vi "Top Level FPGA_w8randLED.vi"() -> ()   [LabVIEW 2012]
uses:
  <vilib>/Platform/TimedLoop/XDataNode/timing_clust.ctl
  <vilib>/Platform/TimedLoop/XDataNode/nitl_modes.ctl
  <vilib>/Platform/TimedLoop/XDataNode/wakeup.ctl
  <vilib>/rvi/DataTransferAndStorage/Container/Common/niFpgaContainerMetaDataKey.ctl
  <vilib>/rvi/DataTransferAndStorage/Container/Common/niFpgaContainerState.ctl
  <vilib>/rvi/DataTransferAndStorage/Container/Common/niFpgaDataTypeControl.ctl
  <vilib>/rvi/DataTransferAndStorage/Container/Common/niFpgaContainerImplementationControl.ctl
  <vilib>/rvi/DataTransferAndStorage/Container/Common/niFpgaContainerArbitrationOptionsControl.ctl
  <vilib>/rvi/DataTransferAndStorage/Container/Common/niFpgaTransferTypeControl.ctl
  <vilib>/rvi/DataTransferAndStorage/Container/Common/niFpgaContainerInitializationParameters.ctl
  <vilib>/rvi/Memory/Memory_Types/niFpgaMemoryInterfaceConfiguration.ctl
  <vilib>/rvi/FIFO/Fifo_Types/niFpgaFifoControlLogicControl.ctl
  <vilib>/rvi/eio/common/nirviEmuTemplateMethod_errors.vi
  <vilib>/rvi/FIFO/Fifo_Resource/nirvififoEmulationSetSize.vi
  <vilib>/rvi/DataTransferAndStorage/Container/Common/niFpgaContainerGetUniqueNameForEmu.vi
  <vilib>/rvi/Emulation/niFpgaSctlEmulationRegisterWithScheduler.vi
  <vilib>/rvi/DataTransferAndStorage/Container/Common/niFpgaContainerSetEmuInfo.vi
  <vilib>/rvi/eio/common/nirviEmuReportErrorAndStop.vi
  <vilib>/rvi/Emulation/niFpgaSctlEmulationScheduler.vi
  <vilib>/rvi/Emulation/niFpgaSctlEmulationFifoFullMgr.vi
  <vilib>/rvi/errors/niFpgaSetErrorForExecOnDevCompSimple.vi
  <vilib>/rvi/Memory/Memory_Emulation/nirvimemoryEmulationManagerCache_GetValue.vi
  <vilib>/rvi/Memory/Memory_Emulation/niFpgaMemoryEmulationValidateCache.vi
  <vilib>/rvi/Memory/Memory_Emulation/nirvimemoryEmulationManagerCache_InsertValue.vi
  <vilib>/rvi/Memory/Memory_Emulation/nirvimemoryEmulationManagerCache_SetValue.vi
  <vilib>/rvi/Emulation/niFpgaSctlEmulationResourceMgr.vi
  <vilib>/rvi/Memory/Memory_Emulation/niFpgaMemoryEmulationCacheClearOnFirstRun.vi
  <vilib>/rvi/Memory/Memory_Emulation/nirvimemoryEmulationManagerCache_MakeExclusive.vi
  <vilib>/rvi/Memory/Memory_Emulation/nirvimemoryEmulationManagerCache_ReleaseExclusive.vi
  <vilib>/Utility/error.llb/Clear Errors.vi
  <vilib>/eio/EIONode/EIONode.xnode
  <vilib>/rvi/DataTransferAndStorage/Container/XNode/niFpgaContainer.xnode
  <vilib>/rvi/FIFO/Fifo_Resource/nirvififoEmulationClear.vi
  <vilib>/Platform/TimedLoop/XDataNode/XDataNode.xnode
  <vilib>/rvi/LocalResourceManager/LocalResourceManager.xnode
  <vilib>/rvi/FIFO/Fifo_Resource/nirvififoEmulationRead.vi
  <vilib>/rvi/DataTransferAndStorage/Register/Emulation/niFpgaRegisterEmulation.vi
  <vilib>/rvi/Memory/Memory_Emulation/nirvimemoryEmulation.vi
  <vilib>/rvi/FIFO/Fifo_Resource/nirvififoEmulationWrite.vi
  <vilib>/Platform/TimedLoop/XDataNode/XDNodeRunTimeDep.lvlib
panel:
  in  "location":i16(ring) items=["Purdue", "NIKHEF", "Zurich", "???"]
  in  "Testpulse duration (20 ns ticks)":u32
  in  "initial value":u64
  in  "channel 7 on/off":bool
  in  "channel 6 on/off":bool
  in  "channel 5 on/off":bool
  in  "channel 4 on/off":bool
  in  "channel 3 on/off":bool
  in  "channel 1 on/off":bool
  in  "channel 2 on/off":bool
  in  "channel 0 on/off":bool
  out "Timestamp":u64
  in  "Stop FPGA and exit":bool
  out "DMA FIFO Timed Out?":bool
  in  "Testpulser On/Off":bool
  in  "Testpulse Time Delay (20 ns ticks)":u32=15
  in  "circular buffer length":u32=1000
  in  "# of pretrigger":u32=20
  out "IO Module\\Pll Unlocked":bool
  out "IO Module\\ADC Error B":bool
  out "IO Module\\ADC Error A":bool
  out "Init Done":bool
  in  "Trigger 4":i16=4000
  in  "Trigger 5":i16=4000
  in  "Trigger 6":i16=4000
  in  "Trigger 7":i16=4000
  in  "Trigger 2":i16=4000
  in  "Trigger 3":i16=4000
  in  "Trigger 1":i16=4000
  in  "Record Size only data":u32=95
  in  "Trigger 0":i16=4000
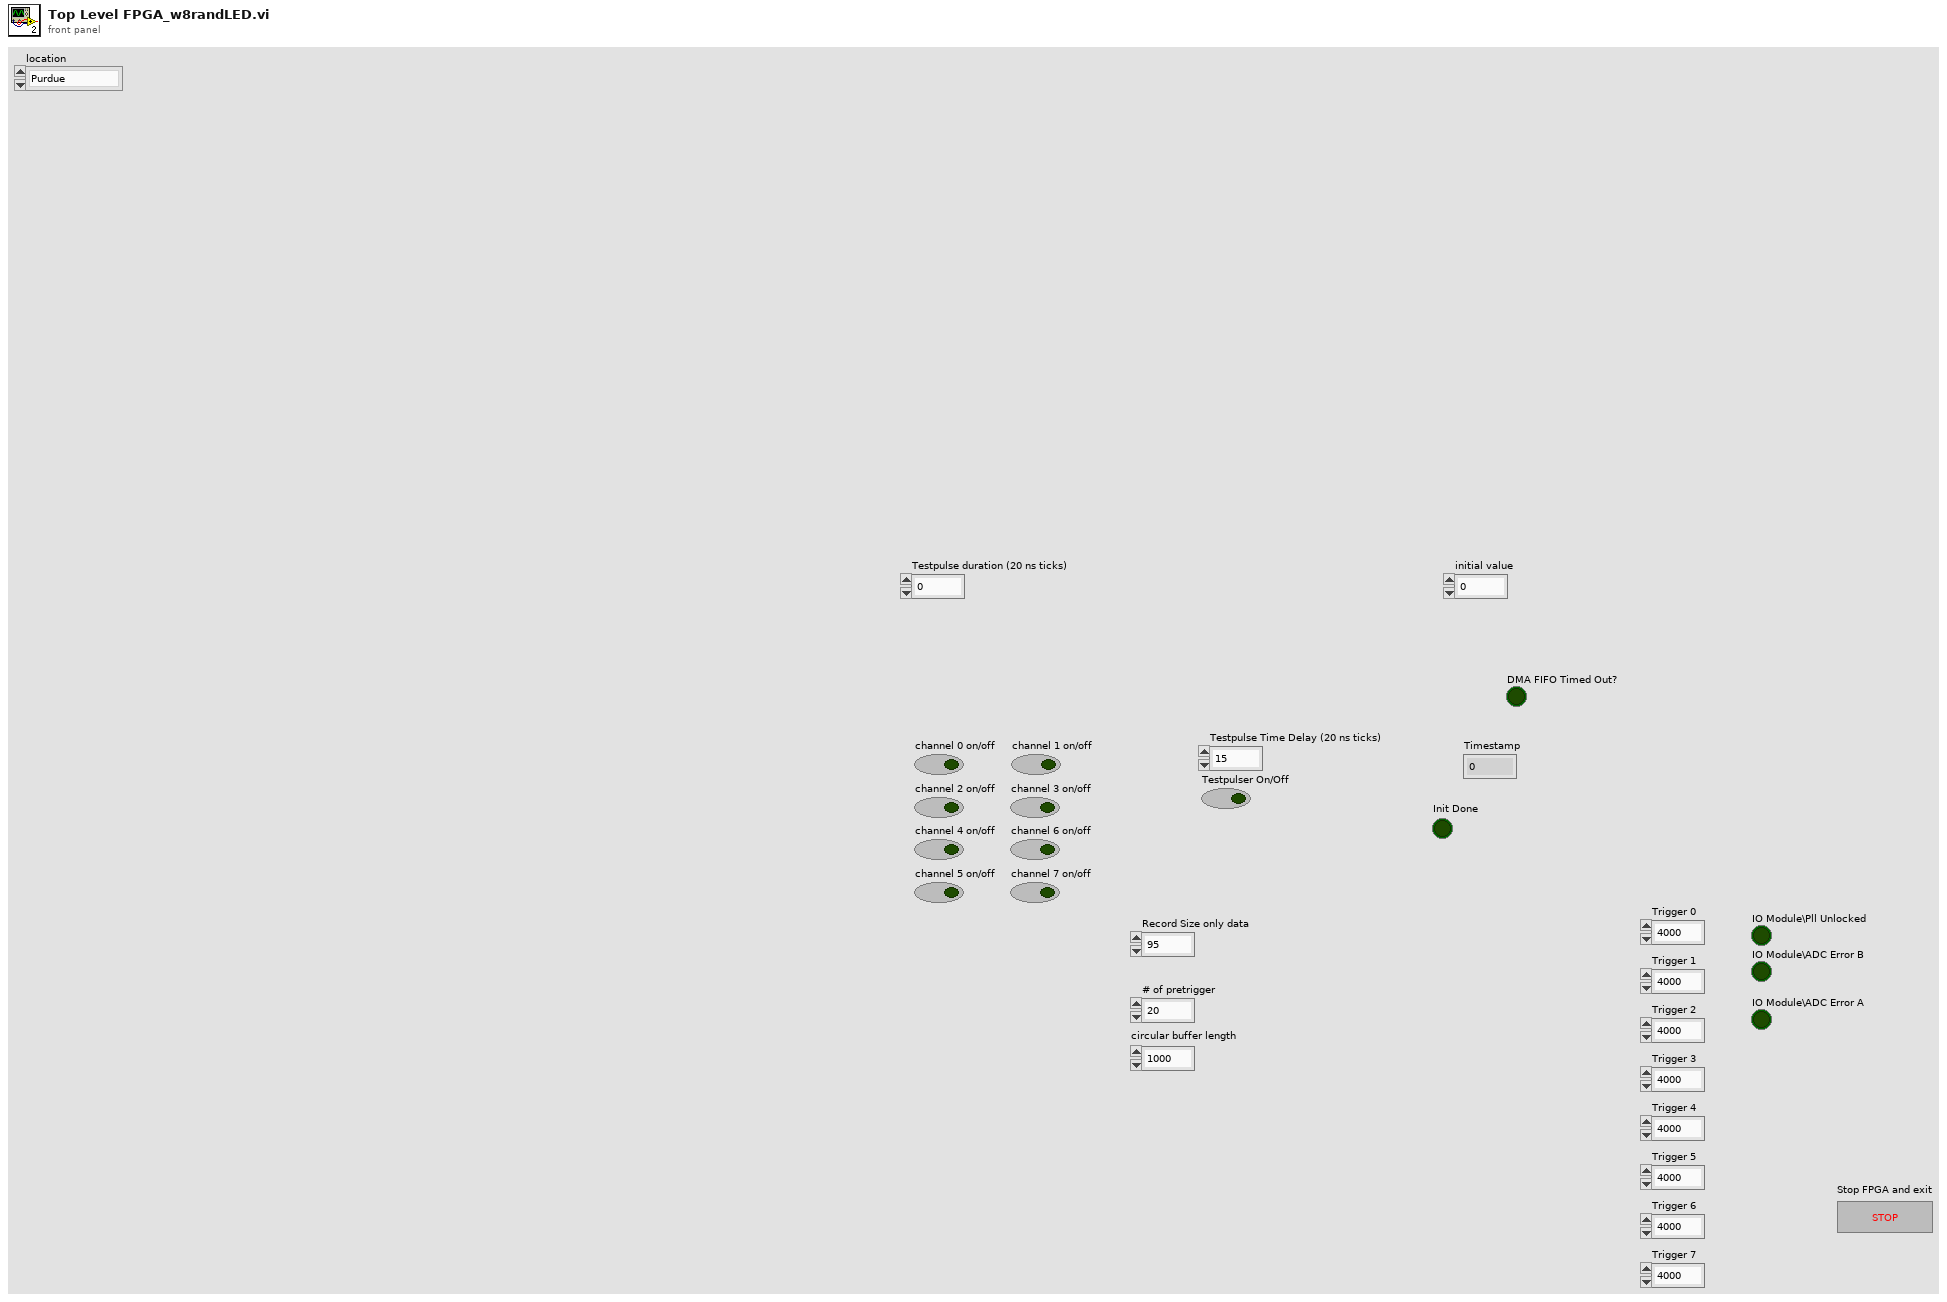
[diagram p1: front panel]
types:
  T1 = typedef "XDNodeRunTimeDep.lvlib/timing_clust.ctl" = cluster{"Expected End [f-1]":u64, "Actual End [f-1]":u64, "Finished Late? [f-1]":bool, "Expected End [i-1]":u64, "Actual End [i-1]":u64, "Finished Late? [i-1]":bool, "Expected Start [i]":u64, "Actual Start [i]":u64, "Expected Start [f]":u64, "Actual Start [f]":u64, "Source Name":string, "Structure Name":string, "Period":i64, "Deadline":i64, "Offset":i64, "Start":i64, "Priority":i32, "Timeout":i32, "Mode":T2, "Wakeup Reason":T3, "Error":errorcluster, "Source Type":string, "Secondary Source Type":string, "Global End Time":u64, "Global Start Time":u64, "Frame Duration":u64, "Iteration Duration":u64, "Assigned CPU":i32, "I/O Scan Engine Mode":u32}
  T2 = typedef "XDNodeRunTimeDep.lvlib/nitl_modes.ctl" = enum32{"No Change", "Process missed periods, maintain original phase", "Discard missed periods, maintain original phase", "Process missed periods, ignore original phase", "Discard missed periods, ignore original phase"}
  T3 = typedef "XDNodeRunTimeDep.lvlib/wakeup.ctl" = enum32{"Normal", "Aborted", "Asynchronous wakeup", "Timing source error", "Timed loop error", "Timeout"}
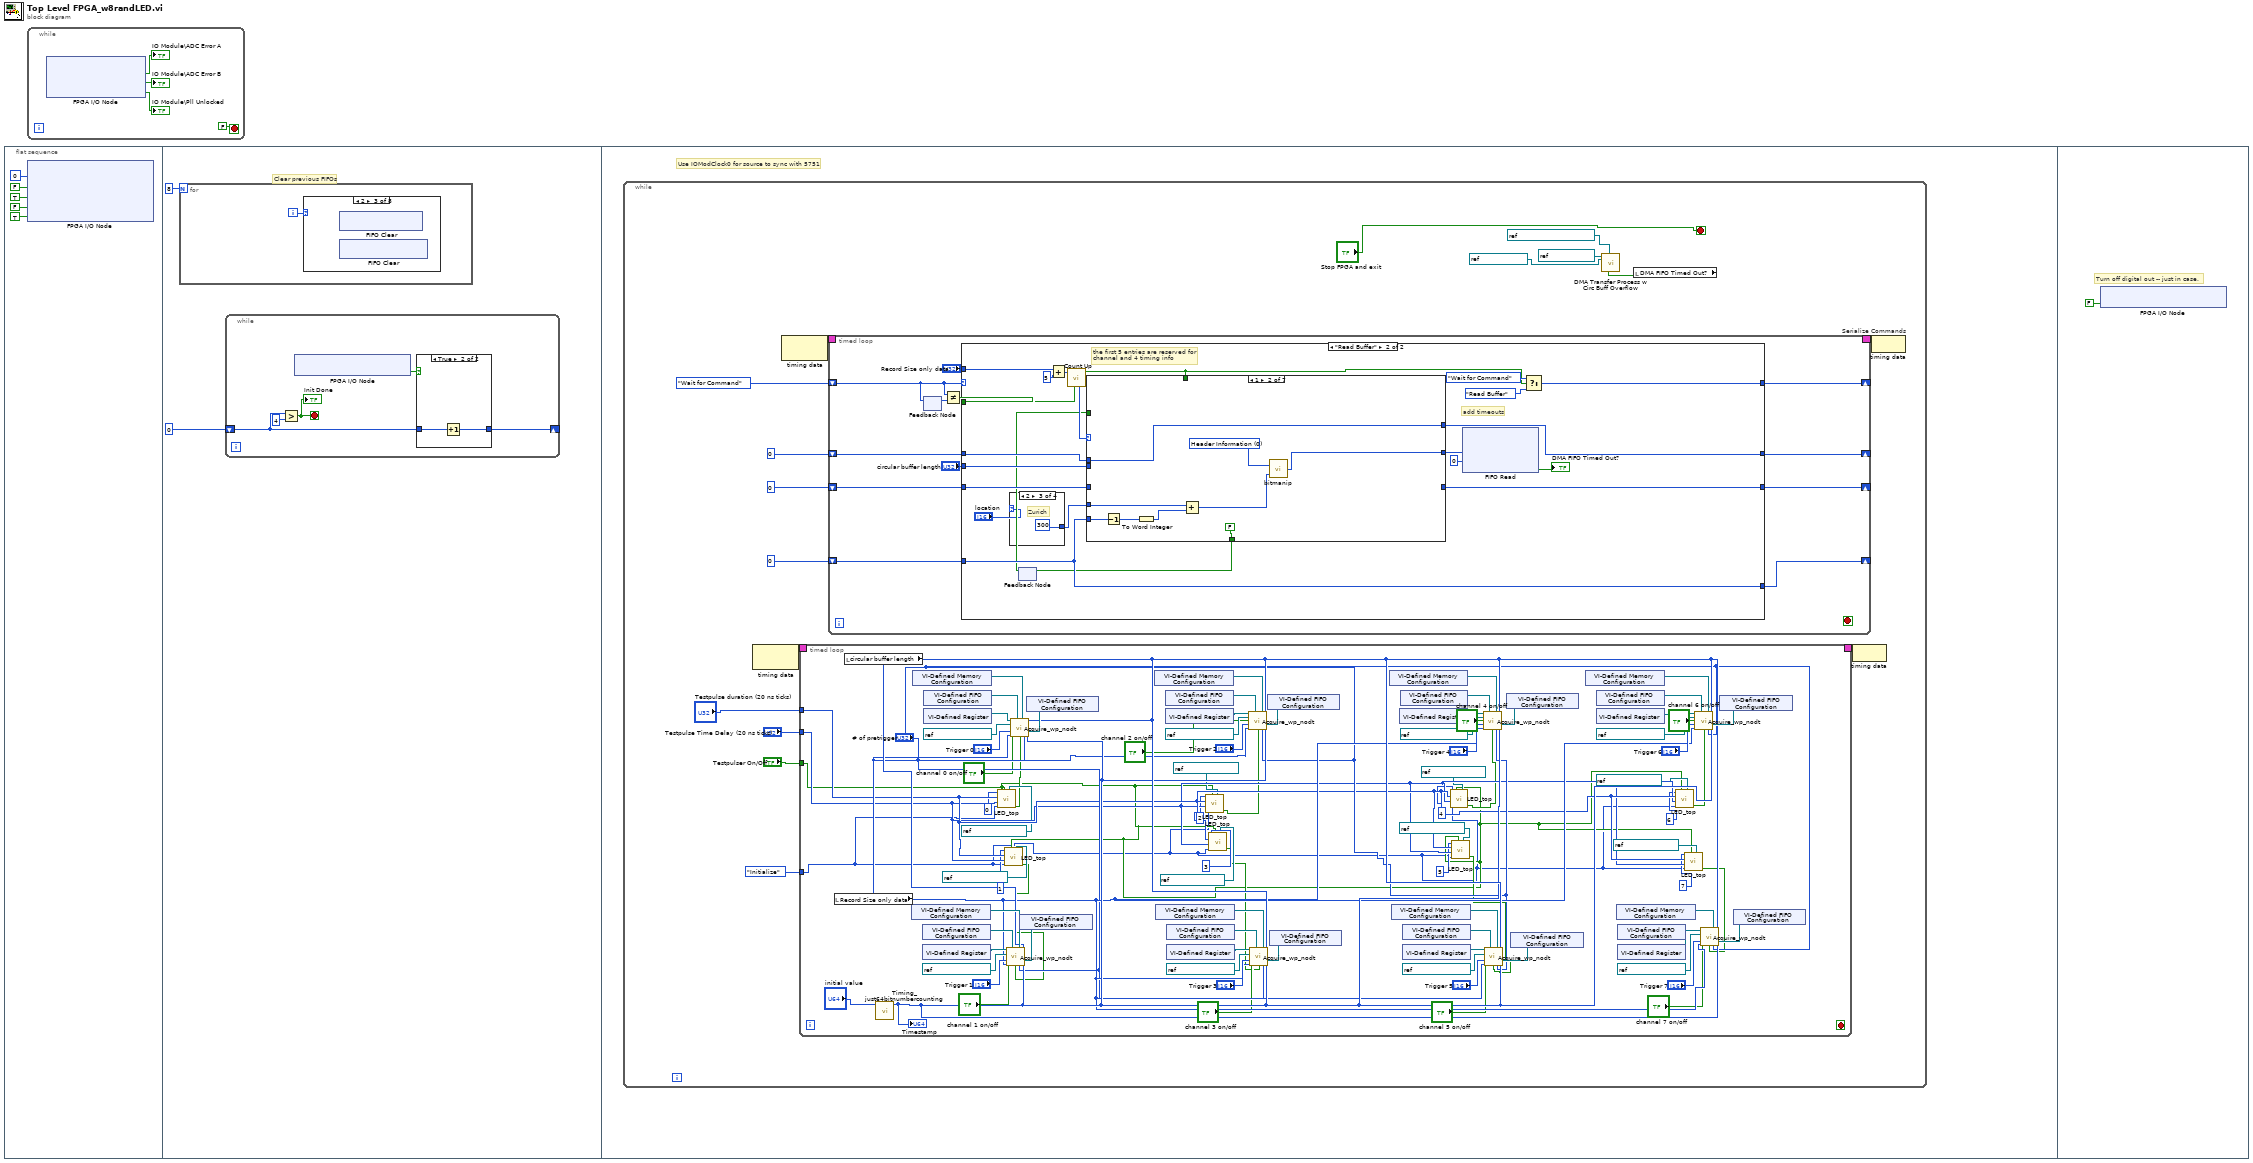
[diagram p0: block diagram]
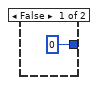
[diagram p2: hidden frame]
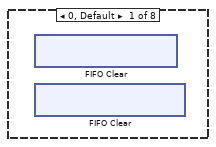
[diagram p3: hidden frame]
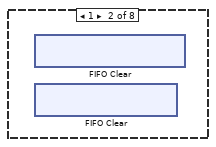
[diagram p4: hidden frame]
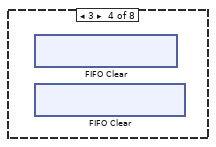
[diagram p5: hidden frame]
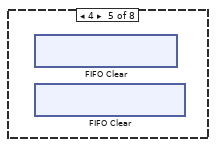
[diagram p6: hidden frame]
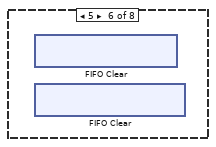
[diagram p7: hidden frame]
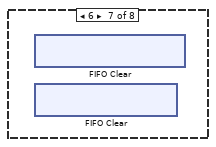
[diagram p8: hidden frame]
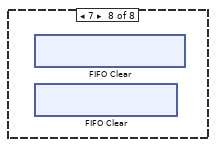
[diagram p9: hidden frame]
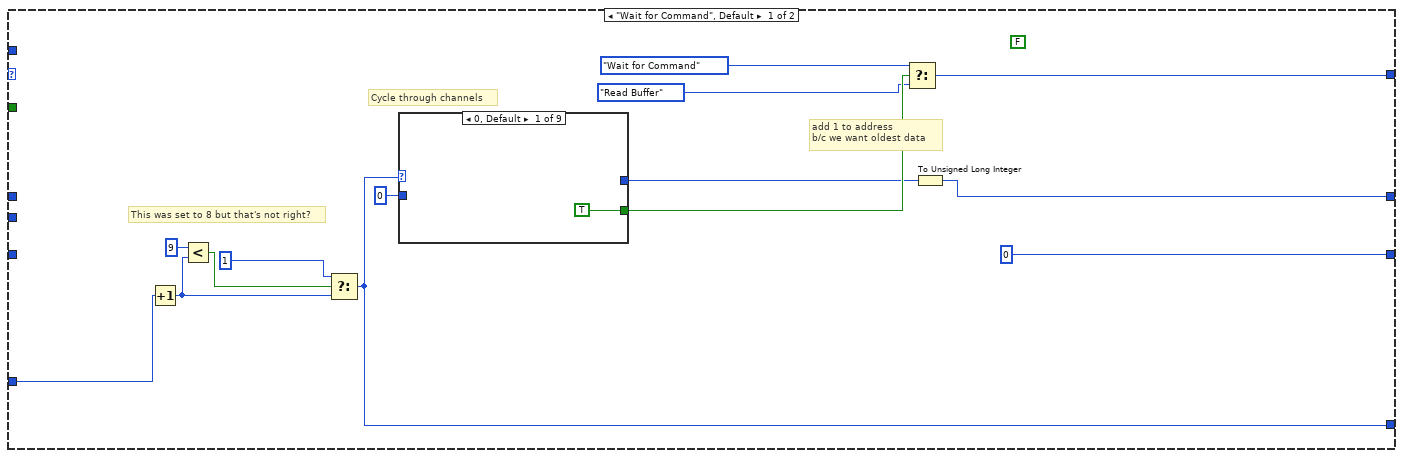
[diagram p10: hidden frame]
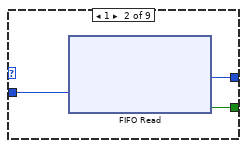
[diagram p11: hidden frame]
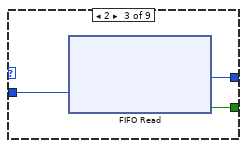
[diagram p12: hidden frame]
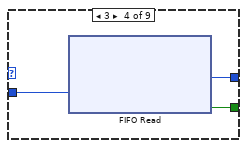
[diagram p13: hidden frame]
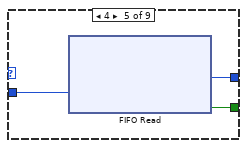
[diagram p14: hidden frame]
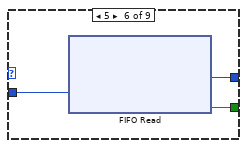
[diagram p15: hidden frame]
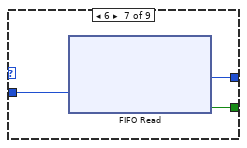
[diagram p16: hidden frame]
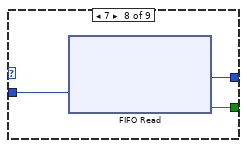
[diagram p17: hidden frame]
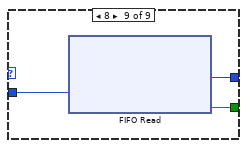
[diagram p18: hidden frame]
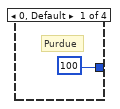
[diagram p19: hidden frame]
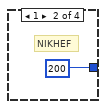
[diagram p20: hidden frame]
diagram:
  n1 = flat-sequence {
    frame #0 {
      n2 = xnode "FPGA I/O Node"("IO Module\\Sample Clock Select"=u8 0 ("IO Module\\Sample Clock Select"), "IO Module\\Force Initialization"=FALSE ("IO Module\\Force Initialization"), "IO Module\\Force Initialization"=TRUE ("IO Module\\Force Initialization"), "IO Module\\Force Initialization"=FALSE ("IO Module\\Force Initialization"), "IO Module\\Digital Output Enable"=TRUE ("IO Module\\Digital Output Enable")) -> ()  [unwired: 5 in, 5 out]
    }
    frame #1 {
      # "Clear previous FIFOs"
      n3 = for {
        N: 8 -> [_]
        i -> [w16]
        n4 = case shown="2" w16 {
          frame 0, Default {
            n5 = xnode ("FIFO Clear")() -> ()  [unwired: 1 in, 1 out]
            n6 = xnode ("FIFO Clear")() -> ()  [unwired: 1 in, 1 out]
          }
          frame 1 {
            n7 = xnode ("FIFO Clear")() -> ()  [unwired: 1 in, 1 out]
            n8 = xnode ("FIFO Clear")() -> ()  [unwired: 1 in, 1 out]
          }
          frame 2 {
            n9 = xnode ("FIFO Clear")() -> ()  [unwired: 1 in, 1 out]
            n10 = xnode ("FIFO Clear")() -> ()  [unwired: 1 in, 1 out]
          }
          frame 3 {
            n11 = xnode ("FIFO Clear")() -> ()  [unwired: 1 in, 1 out]
            n12 = xnode ("FIFO Clear")() -> ()  [unwired: 1 in, 1 out]
          }
          frame 4 {
            n13 = xnode ("FIFO Clear")() -> ()  [unwired: 1 in, 1 out]
            n14 = xnode ("FIFO Clear")() -> ()  [unwired: 1 in, 1 out]
          }
          frame 5 {
            n15 = xnode ("FIFO Clear")() -> ()  [unwired: 1 in, 1 out]
            n16 = xnode ("FIFO Clear")() -> ()  [unwired: 1 in, 1 out]
          }
          frame 6 {
            n17 = xnode ("FIFO Clear")() -> ()  [unwired: 1 in, 1 out]
            n18 = xnode ("FIFO Clear")() -> ()  [unwired: 1 in, 1 out]
          }
          frame 7 {
            n19 = xnode ("FIFO Clear")() -> ()  [unwired: 1 in, 1 out]
            n20 = xnode ("FIFO Clear")() -> ()  [unwired: 1 in, 1 out]
          }
        }
      }
      n21 = while {
        shift-right: [w11] -> _
        shift-left: u16 0 -> [w10]
        stop <- w8 stop-if-true
        n22 = Greater?(x=w10, y=u16 4) -> (0:w8:bool)
        "Init Done" <- w8
        n23 = xnode "FPGA I/O Node"() -> ("IO Module\\Initialization Done"=w12:bool)  [unwired: 1 in, 1 out]
        n24 = case shown="True" w12 {
          tunnel: [u16 0 w15] -> w11
          tunnel: w10 -> [_ w14]
          frame False {
          }
          frame True {
            n25 = Increment(x=w14) -> (x+1=w15:u16)
          }
        }
      }
    }
    frame #2 {
      # "Use IOModClock0 for source to sync with 5751"
      n26 = while {
        stop <- "Stop FPGA and exit" stop-if-true
        n27 = node-c288() -> (w26:T1)  [unwired: 1 in]
        n28 = node-c288() -> (w28:T1)  [unwired: 1 in]
        n29 = timed-loop {
          timing: w26 -> [_]
          timing-out: [_] -> w25
          tunnel: "Testpulser On/Off" -> [w35]
          tunnel: "Testpulse Time Delay (20 ns ticks)" -> [w69]
          tunnel: "Testpulse duration (20 ns ticks)" -> [w70]
          tunnel: enum16{"Initialize", "Get New Value", "Wait"}."Initialize" ("State In") -> [w34]
          stop <- _ stop-if-true
          n30 = local read "Record Size only data"() -> (w73:u32)
          n31 = local read "circular buffer length"() -> (w75:u32)
          n32 = call "Timing_just64bitnumbercounting.vi"("initial value"="initial value") -> ("x+1"=w74:u64)  [unwired: 10 in]
          "Timestamp" <- w74
          n33 = xnode "VI-Defined Memory Configuration"() -> ("Memory Out"=w121:refnum<k21>)
          n34 = xnode "VI-Defined Memory Configuration"() -> ("Memory Out"=w76:refnum<k21>)
          n35 = xnode "VI-Defined FIFO Configuration"() -> ("FIFO Out"=w120:refnum<k21>)
          n36 = xnode "VI-Defined Register"() -> ("Register Out"=w101:refnum<k21>)
          n37 = xnode "VI-Defined FIFO Configuration"() -> ("FIFO Out"=w77:refnum<k21>)
          n38 = xnode "VI-Defined Register"() -> ("Register Out"=w72:refnum<k21>)
          n39 = call "LED_top.vi"("FPGA I/O In"=refnum<k21> "IO Module\\D0 0", "Testpulser On/Off"=w35, "State In"=w34, "Testpulse Time Delay (20 ns ticks)"=w69, "Testpulse duration (20 ns ticks)"=w70, "Address In"=u16 0 ("Total number of pulses sent")) -> ("Is Test Pulse?"=w43:bool)  [unwired: 4 in, 1 out]
          n40 = call "LED_top.vi"("FPGA I/O In"=refnum<k21> "IO Module\\D0 1", "Testpulser On/Off"=w35, "State In"=w34, "Testpulse Time Delay (20 ns ticks)"=w69, "Testpulse duration (20 ns ticks)"=w70, "Address In"=u16 1) -> ("Is Test Pulse?"=w36:bool)  [unwired: 4 in, 1 out]
          n41 = xnode "VI-Defined FIFO Configuration"() -> ("FIFO Out"=w87:refnum<k21>)
          n42 = call "Acquire_wp_nodt.vi"("Ch Armed Reg"=w101, "Command FIFO"=w120, "Circular Buffer Mem"=w121, "circular buffer length"=w75, "FPGA I/O In"=refnum<k21> "IO Module\\AI A1", "channel on/off"="channel 1 on/off", "Trigger"="Trigger 1", "Timing FIFO"=w87, "Samples to Acquire"=w73, "Is Test Pulse?"=w36, "# of pretrigger"="# of pretrigger", "timing"=w74) -> ()  [unwired: 4 in]
          n43 = xnode "VI-Defined FIFO Configuration"() -> ("FIFO Out"=w80:refnum<k21>)
          n44 = call "Acquire_wp_nodt.vi"("Ch Armed Reg"=w72, "Command FIFO"=w77, "Circular Buffer Mem"=w76, "circular buffer length"=w75, "FPGA I/O In"=refnum<k21> "IO Module\\AI A0", "channel on/off"="channel 0 on/off", "Trigger"="Trigger 0", "Timing FIFO"=w80, "Samples to Acquire"=w73, "Is Test Pulse?"=w43, "# of pretrigger"="# of pretrigger", "timing"=w74) -> ()  [unwired: 4 in]
          n45 = xnode "VI-Defined Memory Configuration"() -> ("Memory Out"=w115:refnum<k21>)
          n46 = xnode "VI-Defined Memory Configuration"() -> ("Memory Out"=w118:refnum<k21>)
          n47 = xnode "VI-Defined FIFO Configuration"() -> ("FIFO Out"=w114:refnum<k21>)
          n48 = xnode "VI-Defined Register"() -> ("Register Out"=w97:refnum<k21>)
          n49 = xnode "VI-Defined FIFO Configuration"() -> ("FIFO Out"=w119:refnum<k21>)
          n50 = xnode "VI-Defined Register"() -> ("Register Out"=w99:refnum<k21>)
          n51 = call "LED_top.vi"("FPGA I/O In"=refnum<k21> "IO Module\\D0 2", "Testpulser On/Off"=w35, "State In"=w34, "Testpulse Time Delay (20 ns ticks)"=w69, "Testpulse duration (20 ns ticks)"=w70, "Address In"=u16 2 ("Total number of pulses sent")) -> ("Is Test Pulse?"=w42:bool)  [unwired: 4 in, 1 out]
          n52 = call "LED_top.vi"("FPGA I/O In"=refnum<k21> "IO Module\\D0 3", "Testpulser On/Off"=w35, "State In"=w34, "Testpulse Time Delay (20 ns ticks)"=w69, "Testpulse duration (20 ns ticks)"=w70, "Address In"=u16 3 ("Total number of pulses sent")) -> ("Is Test Pulse?"=w37:bool)  [unwired: 4 in, 1 out]
          n53 = xnode "VI-Defined FIFO Configuration"() -> ("FIFO Out"=w86:refnum<k21>)
          n54 = call "Acquire_wp_nodt.vi"("Ch Armed Reg"=w97, "Command FIFO"=w114, "Circular Buffer Mem"=w115, "circular buffer length"=w75, "FPGA I/O In"=refnum<k21> "IO Module\\AI A2", "channel on/off"="channel 2 on/off", "Trigger"="Trigger 2", "Timing FIFO"=w86, "Samples to Acquire"=w73, "Is Test Pulse?"=w42, "# of pretrigger"="# of pretrigger", "timing"=w74) -> ()  [unwired: 4 in]
          n55 = xnode "VI-Defined FIFO Configuration"() -> ("FIFO Out"=w85:refnum<k21>)
          n56 = call "Acquire_wp_nodt.vi"("Ch Armed Reg"=w99, "Command FIFO"=w119, "Circular Buffer Mem"=w118, "circular buffer length"=w75, "FPGA I/O In"=refnum<k21> "IO Module\\AI A3", "channel on/off"="channel 3 on/off", "Trigger"="Trigger 3", "Timing FIFO"=w85, "Samples to Acquire"=w73, "Is Test Pulse?"=w37, "# of pretrigger"="# of pretrigger", "timing"=w74) -> ()  [unwired: 4 in]
          n57 = xnode "VI-Defined Memory Configuration"() -> ("Memory Out"=w103:refnum<k21>)
          n58 = xnode "VI-Defined Memory Configuration"() -> ("Memory Out"=w106:refnum<k21>)
          n59 = xnode "VI-Defined Register"() -> ("Register Out"=w91:refnum<k21>)
          n60 = xnode "VI-Defined FIFO Configuration"() -> ("FIFO Out"=w102:refnum<k21>)
          n61 = xnode "VI-Defined FIFO Configuration"() -> ("FIFO Out"=w107:refnum<k21>)
          n62 = xnode "VI-Defined Register"() -> ("Register Out"=w95:refnum<k21>)
          n63 = call "LED_top.vi"("FPGA I/O In"=refnum<k21> "IO Module\\D0 4", "Testpulser On/Off"=w35, "State In"=w34, "Testpulse Time Delay (20 ns ticks)"=w69, "Testpulse duration (20 ns ticks)"=w70, "Address In"=u16 4 ("Total number of pulses sent")) -> ("Is Test Pulse?"=w41:bool)  [unwired: 4 in, 1 out]
          n64 = call "LED_top.vi"("FPGA I/O In"=refnum<k21> "IO Module\\D0 5", "Testpulser On/Off"=w35, "State In"=w34, "Testpulse Time Delay (20 ns ticks)"=w69, "Testpulse duration (20 ns ticks)"=w70, "Address In"=u16 5 ("Total number of pulses sent")) -> ("Is Test Pulse?"=w38:bool)  [unwired: 4 in, 1 out]
          n65 = xnode "VI-Defined FIFO Configuration"() -> ("FIFO Out"=w84:refnum<k21>)
          n66 = call "Acquire_wp_nodt.vi"("Ch Armed Reg"=w91, "Command FIFO"=w102, "Circular Buffer Mem"=w103, "circular buffer length"=w75, "FPGA I/O In"=refnum<k21> "IO Module\\AI A4", "channel on/off"="channel 4 on/off", "Trigger"="Trigger 4", "Timing FIFO"=w84, "Samples to Acquire"=w73, "Is Test Pulse?"=w41, "# of pretrigger"="# of pretrigger", "timing"=w74) -> ()  [unwired: 4 in]
          n67 = xnode "VI-Defined FIFO Configuration"() -> ("FIFO Out"=w83:refnum<k21>)
          n68 = call "Acquire_wp_nodt.vi"("Ch Armed Reg"=w95, "Command FIFO"=w107, "Circular Buffer Mem"=w106, "circular buffer length"=w75, "FPGA I/O In"=refnum<k21> "IO Module\\AI A5", "channel on/off"="channel 5 on/off", "Trigger"="Trigger 5", "Timing FIFO"=w83, "Samples to Acquire"=w73, "Is Test Pulse?"=w38, "# of pretrigger"="# of pretrigger", "timing"=w74) -> ()  [unwired: 4 in]
          n69 = xnode "VI-Defined Memory Configuration"() -> ("Memory Out"=w112:refnum<k21>)
          n70 = xnode "VI-Defined FIFO Configuration"() -> ("FIFO Out"=w113:refnum<k21>)
          n71 = xnode "VI-Defined Register"() -> ("Register Out"=w93:refnum<k21>)
          n72 = xnode "VI-Defined Memory Configuration"() -> ("Memory Out"=w109:refnum<k21>)
          n73 = xnode "VI-Defined FIFO Configuration"() -> ("FIFO Out"=w108:refnum<k21>)
          n74 = xnode "VI-Defined Register"() -> ("Register Out"=w89:refnum<k21>)
          n75 = call "LED_top.vi"("FPGA I/O In"=refnum<k21> "IO Module\\D0 6", "Testpulser On/Off"=w35, "State In"=w34, "Testpulse Time Delay (20 ns ticks)"=w69, "Testpulse duration (20 ns ticks)"=w70, "Address In"=u16 6 ("Total number of pulses sent")) -> ("Is Test Pulse?"=w40:bool)  [unwired: 4 in, 1 out]
          n76 = call "LED_top.vi"("FPGA I/O In"=refnum<k21> "IO Module\\D0 7", "Testpulser On/Off"=w35, "State In"=w34, "Testpulse Time Delay (20 ns ticks)"=w69, "Testpulse duration (20 ns ticks)"=w70, "Address In"=u16 7 ("Total number of pulses sent")) -> ("Is Test Pulse?"=w39:bool)  [unwired: 4 in, 1 out]
          n77 = xnode "VI-Defined FIFO Configuration"() -> ("FIFO Out"=w82:refnum<k21>)
          n78 = call "Acquire_wp_nodt.vi"("Ch Armed Reg"=w93, "Command FIFO"=w113, "Circular Buffer Mem"=w112, "circular buffer length"=w75, "FPGA I/O In"=refnum<k21> "IO Module\\AI A6", "channel on/off"="channel 6 on/off", "Trigger"="Trigger 6", "Timing FIFO"=w82, "Samples to Acquire"=w73, "Is Test Pulse?"=w40, "# of pretrigger"="# of pretrigger", "timing"=w74) -> ()  [unwired: 4 in]
          n79 = xnode "VI-Defined FIFO Configuration"() -> ("FIFO Out"=w81:refnum<k21>)
          n80 = call "Acquire_wp_nodt.vi"("Ch Armed Reg"=w89, "Command FIFO"=w108, "Circular Buffer Mem"=w109, "circular buffer length"=w75, "FPGA I/O In"=refnum<k21> "IO Module\\AI A7", "channel on/off"="channel 7 on/off", "Trigger"="Trigger 7", "Timing FIFO"=w81, "Samples to Acquire"=w73, "Is Test Pulse?"=w39, "# of pretrigger"="# of pretrigger", "timing"=w74) -> ()  [unwired: 4 in]
        }
        n81 = timed-loop "Serialize Commands" {
          timing: w28 -> [_]
          timing-out: [_] -> w27
          shift-right: [w901] -> _
          shift-left: enum16{"Wait for Command", "Read Buffer"}."Wait for Command" -> [w899]
          shift-right: [w905] -> _
          shift-left: u32 0 ("Element") -> [w904]
          shift-right: [w903] -> _
          shift-left: u8 0 ("t") -> [w902]
          shift-right: [w896] -> _
          shift-left: u64 0 ("Element") -> [w895]
          stop <- _ stop-if-true
          n82 = feedback-in #1(w899) -> ()
          n83 = feedback #1() -> (w900:enum16{"Wait for Command", "Read Buffer"})  [unwired: 1 in]
          n84 = Not Equal?(x=w899, y=w900) -> (x != y?=w897:bool)
          n85 = case shown="\"Read Buffer\"" w899 {
            tunnel: "Record Size only data" -> [_ w956]
            tunnel: [w909 w966] -> w903
            tunnel: w902 -> [w911 w966]
            tunnel: [w912 w951] -> w905
            tunnel: w904 -> [_ w965]
            tunnel: [w915 w967] -> w901
            tunnel: "circular buffer length" -> [_ w964]
            tunnel: w897 -> [_ w958]
            tunnel: [u64 0 ("Element") w953] -> w896
            tunnel: w895 -> [_ w952]
            frame "Wait for Command", Default {
              (unwired) FALSE
              # "This was set to 8 but that's not right?"
              # "add 1 to address\nb/c we want oldest data"
              # "Cycle through channels"
              n86 = Increment(x=w911) -> (x+1=w910:u8)
              n87 = Less?(x=u8 9, y=w910) -> (x < y?=w919:bool)
              n88 = Select(t=u8 1, s=w919, f=w910) -> (s? t:f=w909:u8)
              n89 = case shown="0, Default" w909 {
                tunnel: [TRUE ("Timed Out?") w924 w925 w928 w931 w934 w937 w940 w943] -> w916
                tunnel: 0 ("Timeout") -> [_ w923 w927 w930 w933 w936 w939 w942 w945]
                tunnel: [_ w922 w926 w929 w932 w935 w938 w941 w944] -> w908
                frame 0, Default {
                }
                frame 1 {
                  n90 = xnode ("FIFO Read")("Timeout"=w923) -> ("Element"=w922:i16, "Timed Out?"=w924:bool)  [unwired: 1 in, 1 out]
                }
                frame 2 {
                  n91 = xnode ("FIFO Read")("Timeout"=w927) -> ("Element"=w926:i16, "Timed Out?"=w925:bool)  [unwired: 1 in, 1 out]
                }
                frame 3 {
                  n92 = xnode ("FIFO Read")("Timeout"=w930) -> ("Element"=w929:i16, "Timed Out?"=w928:bool)  [unwired: 1 in, 1 out]
                }
                frame 4 {
                  n93 = xnode ("FIFO Read")("Timeout"=w933) -> ("Element"=w932:i16, "Timed Out?"=w931:bool)  [unwired: 1 in, 1 out]
                }
                frame 5 {
                  n94 = xnode ("FIFO Read")("Timeout"=w936) -> ("Element"=w935:i16, "Timed Out?"=w934:bool)  [unwired: 1 in, 1 out]
                }
                frame 6 {
                  n95 = xnode ("FIFO Read")("Timeout"=w939) -> ("Element"=w938:i16, "Timed Out?"=w937:bool)  [unwired: 1 in, 1 out]
                }
                frame 7 {
                  n96 = xnode ("FIFO Read")("Timeout"=w942) -> ("Element"=w941:i16, "Timed Out?"=w940:bool)  [unwired: 1 in, 1 out]
                }
                frame 8 {
                  n97 = xnode ("FIFO Read")("Timeout"=w945) -> ("Element"=w944:i16, "Timed Out?"=w943:bool)  [unwired: 1 in, 1 out]
                }
              }
              n98 = Select(t=enum16{"Wait for Command", "Read Buffer"}."Wait for Command", s=w916, f=enum16{"Wait for Command", "Read Buffer"}."Read Buffer") -> (s? t:f=w915:enum16{"Wait for Command", "Read Buffer"})
              n99 = To Unsigned Long Integer(number=w908) -> (unsigned 32bit integer=w912:u32)
            }
            frame "Read Buffer" {
              # "the first 5 entries are reserved for channel and 4 timing info"
              # "add timeouts"
              n100 = case shown="2" "location" {
                tunnel: [i16 100 i16 200 i16 300 i16 400] -> w946
                frame 0, Default {
                  # "Purdue"
                }
                frame 1 {
                  # "NIKHEF"
                }
                frame 2 {
                  # "Zurich"
                }
                frame 3 {
                  # "???"
                }
              }
              n101 = feedback #2() -> (w950:bool)  [unwired: 1 in]
              n102 = Add(x=w956, y=u32 5) -> (x+y=w954:u32)
              n103 = call "Count Up.vi"("Reset?"=w958, "goal"=w954) -> ("Count Met"=w960:bool, "count"=w957:u32)  [unwired: 8 in]
              n104 = case shown="1" w957 {
                tunnel: w966 -> [_ w979 w987 _ _ _ w1026]
                tunnel: w965 -> [_ w984 w989 w1010 w1016 w1022 w1033]
                tunnel: w964 -> [_ _ _ _ _ _ w1032]
                tunnel: w960 -> [_ _ _ _ _ _ w1031]
                tunnel: [i16 0 ("Data") w982 w991 w1008 w1014 w1020 w1027] -> w959
                tunnel: w950 -> [_ _ _ _ _ _ w1029]
                tunnel: [u64 0 ("Element") _ w988 w1011 w1017 w1023 _] -> w953
                tunnel: w952 -> [_ _ _ w1011 w1017 w1023 _]
                tunnel: [u32 0 ("Element") w984 w989 w1010 w1016 w1022 _] -> w951
                tunnel: [FALSE FALSE FALSE FALSE FALSE TRUE FALSE] -> w949
                tunnel: w946 -> [_ w977 _ _ _ _ _]
                frame 0, Default {
                }
                frame 1 {
                  w981 = u16 0 items=["Header Information", "Particle Pulse", "Test Pulse"] ("Pulse Type")
                  n105 = Decrement(x=w979) -> (x-1=w980:u8)
                  n106 = To Word Integer(number=w980) -> (16bit integer=w978:i16)
                  n107 = Add(x=w977, y=w978) -> (x+y=w976:i16)
                  n108 = call "bitmanip.vi"("Pulse Type"=w981, "Integer to be written"=w976) -> ("Integer Written"=w982:i16)  [unwired: 2 in]
                }
                frame 2 {
                  # "reads out the lsb of the timing information"
                  n109 = case shown="2" w987 {
                    tunnel: [_ w992 w994 w996 w998 w1000 w1002 w1004 w1006] -> w988
                    frame Default {
                    }
                    frame 1 {
                      n110 = xnode ("FIFO Read")("Timeout"=0) -> ("Element"=w992:u64)  [unwired: 1 in, 2 out]
                    }
                    frame 2 {
                      n111 = xnode ("FIFO Read")("Timeout"=0) -> ("Element"=w994:u64)  [unwired: 1 in, 2 out]
                    }
                    frame 3 {
                      n112 = xnode ("FIFO Read")("Timeout"=0) -> ("Element"=w996:u64)  [unwired: 1 in, 2 out]
                    }
                    frame 4 {
                      n113 = xnode ("FIFO Read")("Timeout"=0) -> ("Element"=w998:u64)  [unwired: 1 in, 2 out]
                    }
                    frame 5 {
                      n114 = xnode ("FIFO Read")("Timeout"=0) -> ("Element"=w1000:u64)  [unwired: 1 in, 2 out]
                    }
                    frame 6 {
                      n115 = xnode ("FIFO Read")("Timeout"=0) -> ("Element"=w1002:u64)  [unwired: 1 in, 2 out]
                    }
                    frame 7 {
                      n116 = xnode ("FIFO Read")("Timeout"=0) -> ("Element"=w1004:u64)  [unwired: 1 in, 2 out]
                    }
                    frame 8 {
                      n117 = xnode ("FIFO Read")("Timeout"=0) -> ("Element"=w1006:u64)  [unwired: 1 in, 2 out]
                    }
                  }
                  n118 = Split Number(x=w988) -> (hi(x)=w986:u32)  [unwired: 1 out]
                  n119 = Split Number(x=w986) -> (hi(x)=w985:u16)  [unwired: 1 out]
                  n120 = To Word Integer(number=w985) -> (16bit integer=w991:i16)
                }
                frame 3 {
                  n121 = Split Number(x=w1011) -> (hi(x)=w1013:u32)  [unwired: 1 out]
                  n122 = Split Number(x=w1013) -> (lo(x)=w1012:u16)  [unwired: 1 out]
                  n123 = To Word Integer(number=w1012) -> (16bit integer=w1008:i16)
                }
                frame 4 {
                  n124 = Split Number(x=w1017) -> (lo(x)=w1019:u32)  [unwired: 1 out]
                  n125 = Split Number(x=w1019) -> (hi(x)=w1018:u16)  [unwired: 1 out]
                  n126 = To Word Integer(number=w1018) -> (16bit integer=w1014:i16)
                }
                frame 5 {
                  n127 = Split Number(x=w1023) -> (lo(x)=w1025:u32)  [unwired: 1 out]
                  n128 = Split Number(x=w1025) -> (lo(x)=w1024:u16)  [unwired: 1 out]
                  n129 = To Word Integer(number=w1024) -> (16bit integer=w1020:i16)
                }
                frame 6.. {
                  n130 = call "Circular Buffer Address_try_without_deadtime.vi"("Reset?"=w1029, "Starting Address"=w1033, "circular buffer length"=w1032) -> ("Address"=w1030:u32)  [unwired: 8 in]
                  n131 = case shown="1" w1026 {
                    tunnel: w1030 -> [_ w1037 w1040 w1043 w1046 w1049 w1052 w1055 w1058]
                    tunnel: w1031 -> [_ w1036 w1039 w1042 w1045 w1048 w1051 w1054 w1057]
                    tunnel: [i16 0 w1035 w1038 w1041 w1044 w1047 w1050 w1053 w1056] -> w1027
                    frame Default {
                      # "Error"
                    }
                    frame 1 {
                      n132 = xnode ("Memory Read")("Address"=w1037) -> ("Data"=w1035:i16)  [unwired: 1 in, 1 out]
                      n133 = xnode ("Register Write")("Data"=w1036) -> ()  [unwired: 1 in, 1 out]
                    }
                    frame 2 {
                      n134 = xnode ("Memory Read")("Address"=w1040) -> ("Data"=w1038:i16)  [unwired: 1 in, 1 out]
                      n135 = xnode ("Register Write")("Data"=w1039) -> ()  [unwired: 1 in, 1 out]
                    }
                    frame 3 {
                      n136 = xnode ("Memory Read")("Address"=w1043) -> ("Data"=w1041:i16)  [unwired: 1 in, 1 out]
                      n137 = xnode ("Register Write")("Data"=w1042) -> ()  [unwired: 1 in, 1 out]
                    }
                    frame 4 {
                      n138 = xnode ("Memory Read")("Address"=w1046) -> ("Data"=w1044:i16)  [unwired: 1 in, 1 out]
                      n139 = xnode ("Register Write")("Data"=w1045) -> ()  [unwired: 1 in, 1 out]
                    }
                    frame 5 {
                      n140 = xnode ("Memory Read")("Address"=w1049) -> ("Data"=w1047:i16)  [unwired: 1 in, 1 out]
                      n141 = xnode ("Register Write")("Data"=w1048) -> ()  [unwired: 1 in, 1 out]
                    }
                    frame 6 {
                      n142 = xnode ("Memory Read")("Address"=w1052) -> ("Data"=w1050:i16)  [unwired: 1 in, 1 out]
                      n143 = xnode ("Register Write")("Data"=w1051) -> ()  [unwired: 1 in, 1 out]
                    }
                    frame 7 {
                      n144 = xnode ("Memory Read")("Address"=w1055) -> ("Data"=w1053:i16)  [unwired: 1 in, 1 out]
                      n145 = xnode ("Register Write")("Data"=w1054) -> ()  [unwired: 1 in, 1 out]
                    }
                    frame 8 {
                      n146 = xnode ("Memory Read")("Address"=w1058) -> ("Data"=w1056:i16)  [unwired: 1 in, 1 out]
                      n147 = xnode ("Register Write")("Data"=w1057) -> ()  [unwired: 1 in, 1 out]
                    }
                  }
                }
              }
              n148 = feedback-in #2(w949) -> ()
              n149 = xnode ("FIFO Read")("Element"=w959, "Timeout"=0) -> ("Timed Out?"=→"DMA FIFO Timed Out?":bool)  [unwired: 1 in, 1 out]
              n150 = Select(t=enum16{"Wait for Command", "Read Buffer"}."Wait for Command", s=w960, f=enum16{"Wait for Command", "Read Buffer"}."Read Buffer") -> (s? t:f=w967:enum16{"Wait for Command", "Read Buffer"})
            }
          }
        }
        n151 = local read "DMA FIFO Timed Out?"() -> (w31:bool)
        n152 = call "DMA Transfer Process w Circ Buff Overflow.vi"("DMA Write Timed Out?"=w31, "Clock Domain"=refnum<k21> "40 MHz Onboard Clock", "Local"=refnum<k21> "To DMA FIFO", "DMA"=refnum<k21> "To Host FIFO") -> ()  [unwired: 8 in]
        n153 = node-c288(w25) -> ()
        n154 = node-c288(w27) -> ()
      }
    }
    frame #3 {
      # "Turn off digital out -- just in case."
      n155 = xnode "FPGA I/O Node"("IO Module\\Digital Output Enable"=FALSE ("IO Module\\Digital Output Enable")) -> ()  [unwired: 1 in, 1 out]
    }
  }
  n156 = while {
    stop <- FALSE stop-if-true
    n157 = xnode "FPGA I/O Node"() -> ("IO Module\\ADC Error A"=→"IO Module\\ADC Error A":bool, "IO Module\\ADC Error B"=→"IO Module\\ADC Error B":bool, "IO Module\\Pll Unlocked"=→"IO Module\\Pll Unlocked":bool)  [unwired: 3 in, 3 out]
  }
